vi "Spinner2.vi"(5 "String In":string="sweeping") -> (2 "Spinner Out":string)   [LabVIEW 2019, in "Instrument.Lockin.lvlib" / "Instrument UI.Lockin.lvclass"]
uses:
  Instrument UI.Lockin.lvclass
  8a7dd14e-c393-41ec-a15c-c489bce8c11d.vi
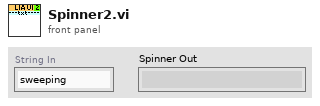
[diagram p1: front panel]
types:
  T1 = enum32{"Bad", "Idle", "Run top level", "Running"}
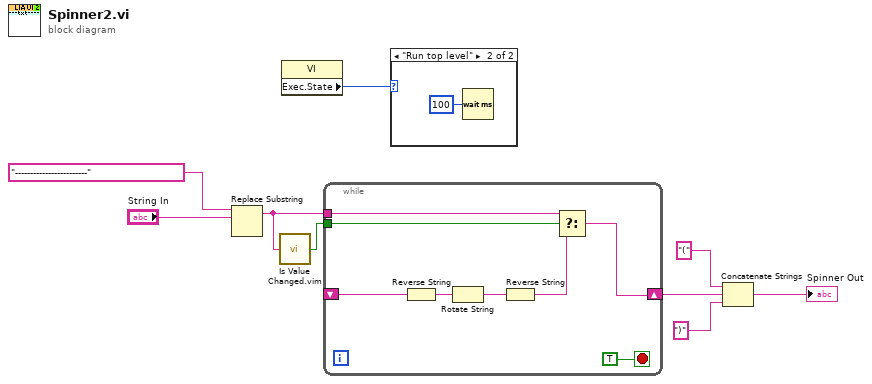
[diagram p0: block diagram]
diagram:
  n1 = Replace Substring(4:"String In", 5:"------------------------") -> (1:w1:string)  [unwired: 2 in, 1 out]
  n2 = call "Is Value Changed.vim"("value"=w1) -> ("changed or first call?"=w3:bool)
  n3 = property class="VI"() -> ("Exec.State"=w9:T1)  [unwired: 2 in, 2 out]
  n4 = while {
    shift-right: [w16] -> w8
    shift-left: _ -> [w14]
    tunnel: w1 -> [w13]
    tunnel: w3 -> [w10]
    stop <- TRUE stop-if-true
    n5 = Reverse String(1:w14) -> (0:w12:string)
    n6 = Rotate String(1:w12) -> (0:w11:string)
    n7 = Reverse String(1:w11) -> (0:w15:string)
    n8 = Select(t=w13, s=w10, f=w15) -> (s? t:f=w16:string)
  }
  n9 = case shown="\"Run top level\"" w9 {
    frame Default {
    }
    frame "Run top level" {
      n10 = Wait (ms)(milliseconds to wait=u32 100) -> ()  [unwired: 1 out]
    }
  }
  n11 = Concatenate Strings("(", w8, ")") -> (→"Spinner Out":string)
